vi "GUI_HTU_BCavePhosphors.vi"() -> ()   [LabVIEW 2020]
uses:
  Shared/GUI_Template/GUI_master/tcp_new_data_event.ctl
  Shared/GUI_Template/GUI_master/tcp new data cluster.ctl
  General GUIs/Device GUIs/GUI_Cameras/Controls/Crosshair type def.ctl
  <userlib>/_OpenG.lib/array/array.llb/Filter 1D Array with Scalar (String)__ogtk.vi
panel:
  in  "GUIdevice 8":string="U_PLC"
  in  "Position.Channel 8::7":T1(ring) caption="TC phosphor"
  in  "GUIdevice 7":string="U_1WireBcave"
  in  "DO.Ch4::8":enum16{"on", "off"}(ring) caption="Phosphor1"
  in  "DO.Ch2::8":enum16{"on", "off"}(ring) caption="Chicane Slits"
  in  "DigitalOutput.Channel 1::6":enum16{"on", "off"}(ring) caption="DC Phosphor"
  in  "GUIdevice 6":string="U_Valve_Daq"
  out "String 4":string="x1\ny1\nx2\ny2"
  out "String 3":string="x1\ny1\nx2\ny2"
  out "String 2":string="x1\ny1\nx2\ny2"
  out "String":string="x1\ny1\nx2\ny2"
  in  "visibility":bool=TRUE
  out "appended array":string[](array[string]) caption="XH"
  out "appended array 6":string[](array[string]) caption="XH"
  out "appended array 8":string[](array[string]) caption="XH"
  out "appended array 4":string[](array[string]) caption="XH"
  in  "UDP error message":string
  out "tcp data event 2":T2
  out "error IO 2":errorcluster
  in  "Color Box":u32(colorbox)
  in  "TargetSize.Y::5":dbl=45.0 caption="y" min=2.0 max=3000.0 format="%#_6f"
  in  "TargetSize.X::5":dbl=47.0 caption="x" min=2.0 max=3000.0 format="%#_6f"
  in  "TargetSize.Y::4":dbl=45.0 caption="y" min=2.0 max=3000.0 format="%#_6f"
  in  "TargetSize.X::4":dbl=47.0 caption="x" min=2.0 max=3000.0 format="%#_6f"
  in  "TargetSize.Y::3":dbl=163.0 caption="y" min=2.0 max=3000.0 format="%#_6f"
  in  "TargetSize.X::3":dbl=152.0 caption="x" min=2.0 max=3000.0 format="%#_6f"
  in  "TargetSize.Y::2":dbl=74.0 caption="y" min=2.0 max=3000.0 format="%#_6f"
  in  "TargetSize.X::2":dbl=75.0 caption="x" min=2.0 max=3000.0 format="%#_6f"
  in  "active cams":string
  out "CCDs":string[](array[string])
  out "Cameras":T3
  in  "Target.Y::5":dbl=45.0 caption="y" min=0.0 max=2000.0 format="%#_6f"
  in  "Target.X::5":dbl=47.0 caption="x" min=0.0 max=2000.0 format="%#_6f"
  in  "Target.Y::4":dbl=45.0 caption="y" min=0.0 max=2000.0 format="%#_6f"
  in  "Target.X::4":dbl=47.0 caption="x" min=0.0 max=2000.0 format="%#_6f"
  in  "Target.Y::3":dbl=163.0 caption="y" min=0.0 max=2000.0 format="%#_6f"
  in  "Target.X::3":dbl=152.0 caption="x" min=0.0 max=2000.0 format="%#_6f"
  in  "Target.Y::2":dbl=74.0 caption="y" min=0.0 max=2000.0 format="%#_6f"
  in  "Target.X::2":dbl=75.0 caption="x" min=0.0 max=2000.0 format="%#_6f"
  out "error out":errorcluster
  in  "triggerdelay::5":dbl=0.001 caption="triggerdelay" min=0.0 max=50000.0 format="%_4p"
  in  "triggerdelay::4":dbl=0.001 caption="triggerdelay" min=0.0 max=50000.0 format="%_4p"
  in  "triggerdelay::3":dbl=0.001 caption="triggerdelay" min=15.0 max=1000000.0 format="%_4p"
  in  "triggerdelay::2":dbl=0.001 caption="triggerdelay" min=500.0 max=1000000.0 format="%_4p"
  in  "trigger::5":bool caption="Trigger"
  in  "centroidy::5":dbl=0.001 caption="centroid y" min=0.0 max=0.0 format="%_4f"
  in  "centroidx::5":dbl=0.001 caption="centroid x" min=0.0 max=0.0 format="%_4f"
  in  "exposure::5":dbl=0.001 caption="exposure" min=0.0001 max=1.0 format="%_4p"
  out "image::5":T4(plugin-control) caption="HTT-MagCam-01"
  in  "GUIdevice 5":string="UC_Phosphor1"
  in  "trigger::4":bool caption="Trigger"
  in  "centroidy::4":dbl=0.001 caption="centroid y" min=0.0 max=0.0 format="%_4f"
  in  "centroidx::4":dbl=0.001 caption="centroid x" min=0.0 max=0.0 format="%_4f"
  in  "exposure::4":dbl=0.001 caption="exposure" min=0.0001 max=1.0 format="%_4p"
  out "image::4":T4(plugin-control) caption="HTT-MagCam-02"
  in  "GUIdevice 4":string="UC_DiagnosticsPhosphor"
  in  "trigger::3":bool caption="Trigger"
  in  "centroidy::3":dbl=0.001 caption="centroid y" min=0.0 max=0.0 format="%_4f"
  in  "centroidx::3":dbl=0.001 caption="centroid x" min=0.0 max=0.0 format="%_4f"
  in  "exposure::3":dbl=0.001 caption="exposure" min=2e-05 max=1.0 format="%_4p"
  out "image::3":T4(plugin-control) caption="HTT-MagCam-03"
  in  "GUIdevice 3":string="UC_ChicaneSlit"
  in  "trigger::2":bool caption="Trigger"
  in  "centroidy::2":dbl=0.001 caption="centroid y" min=0.0 max=0.0 format="%_4f"
  in  "centroidx::2":dbl=0.001 caption="centroid x" min=0.0 max=0.0 format="%_4f"
  in  "exposure::2":dbl=0.001 caption="exposure" min=2e-05 max=1.0 format="%_4p"
  out "image::2":T4(plugin-control) caption="HTT-MagCam-04"
  in  "GUIdevice 2":string="UC_TC_Phosphor"
  out "tcp data event":T2
  in  "Refresh Button":bool caption="Update Crosshairs"
  in  "Select device":string(combo)="FrogHPD"
  in  "stop":bool
  in  "GUIdevice 1":string="HPD_CCD"
  # "XHair location"
  # "XHair location"
  # "XHair size"
  # "XHair size"
  # "XHair location"
  # "XHair size"
  # "XHair size"
  # "XHair location"
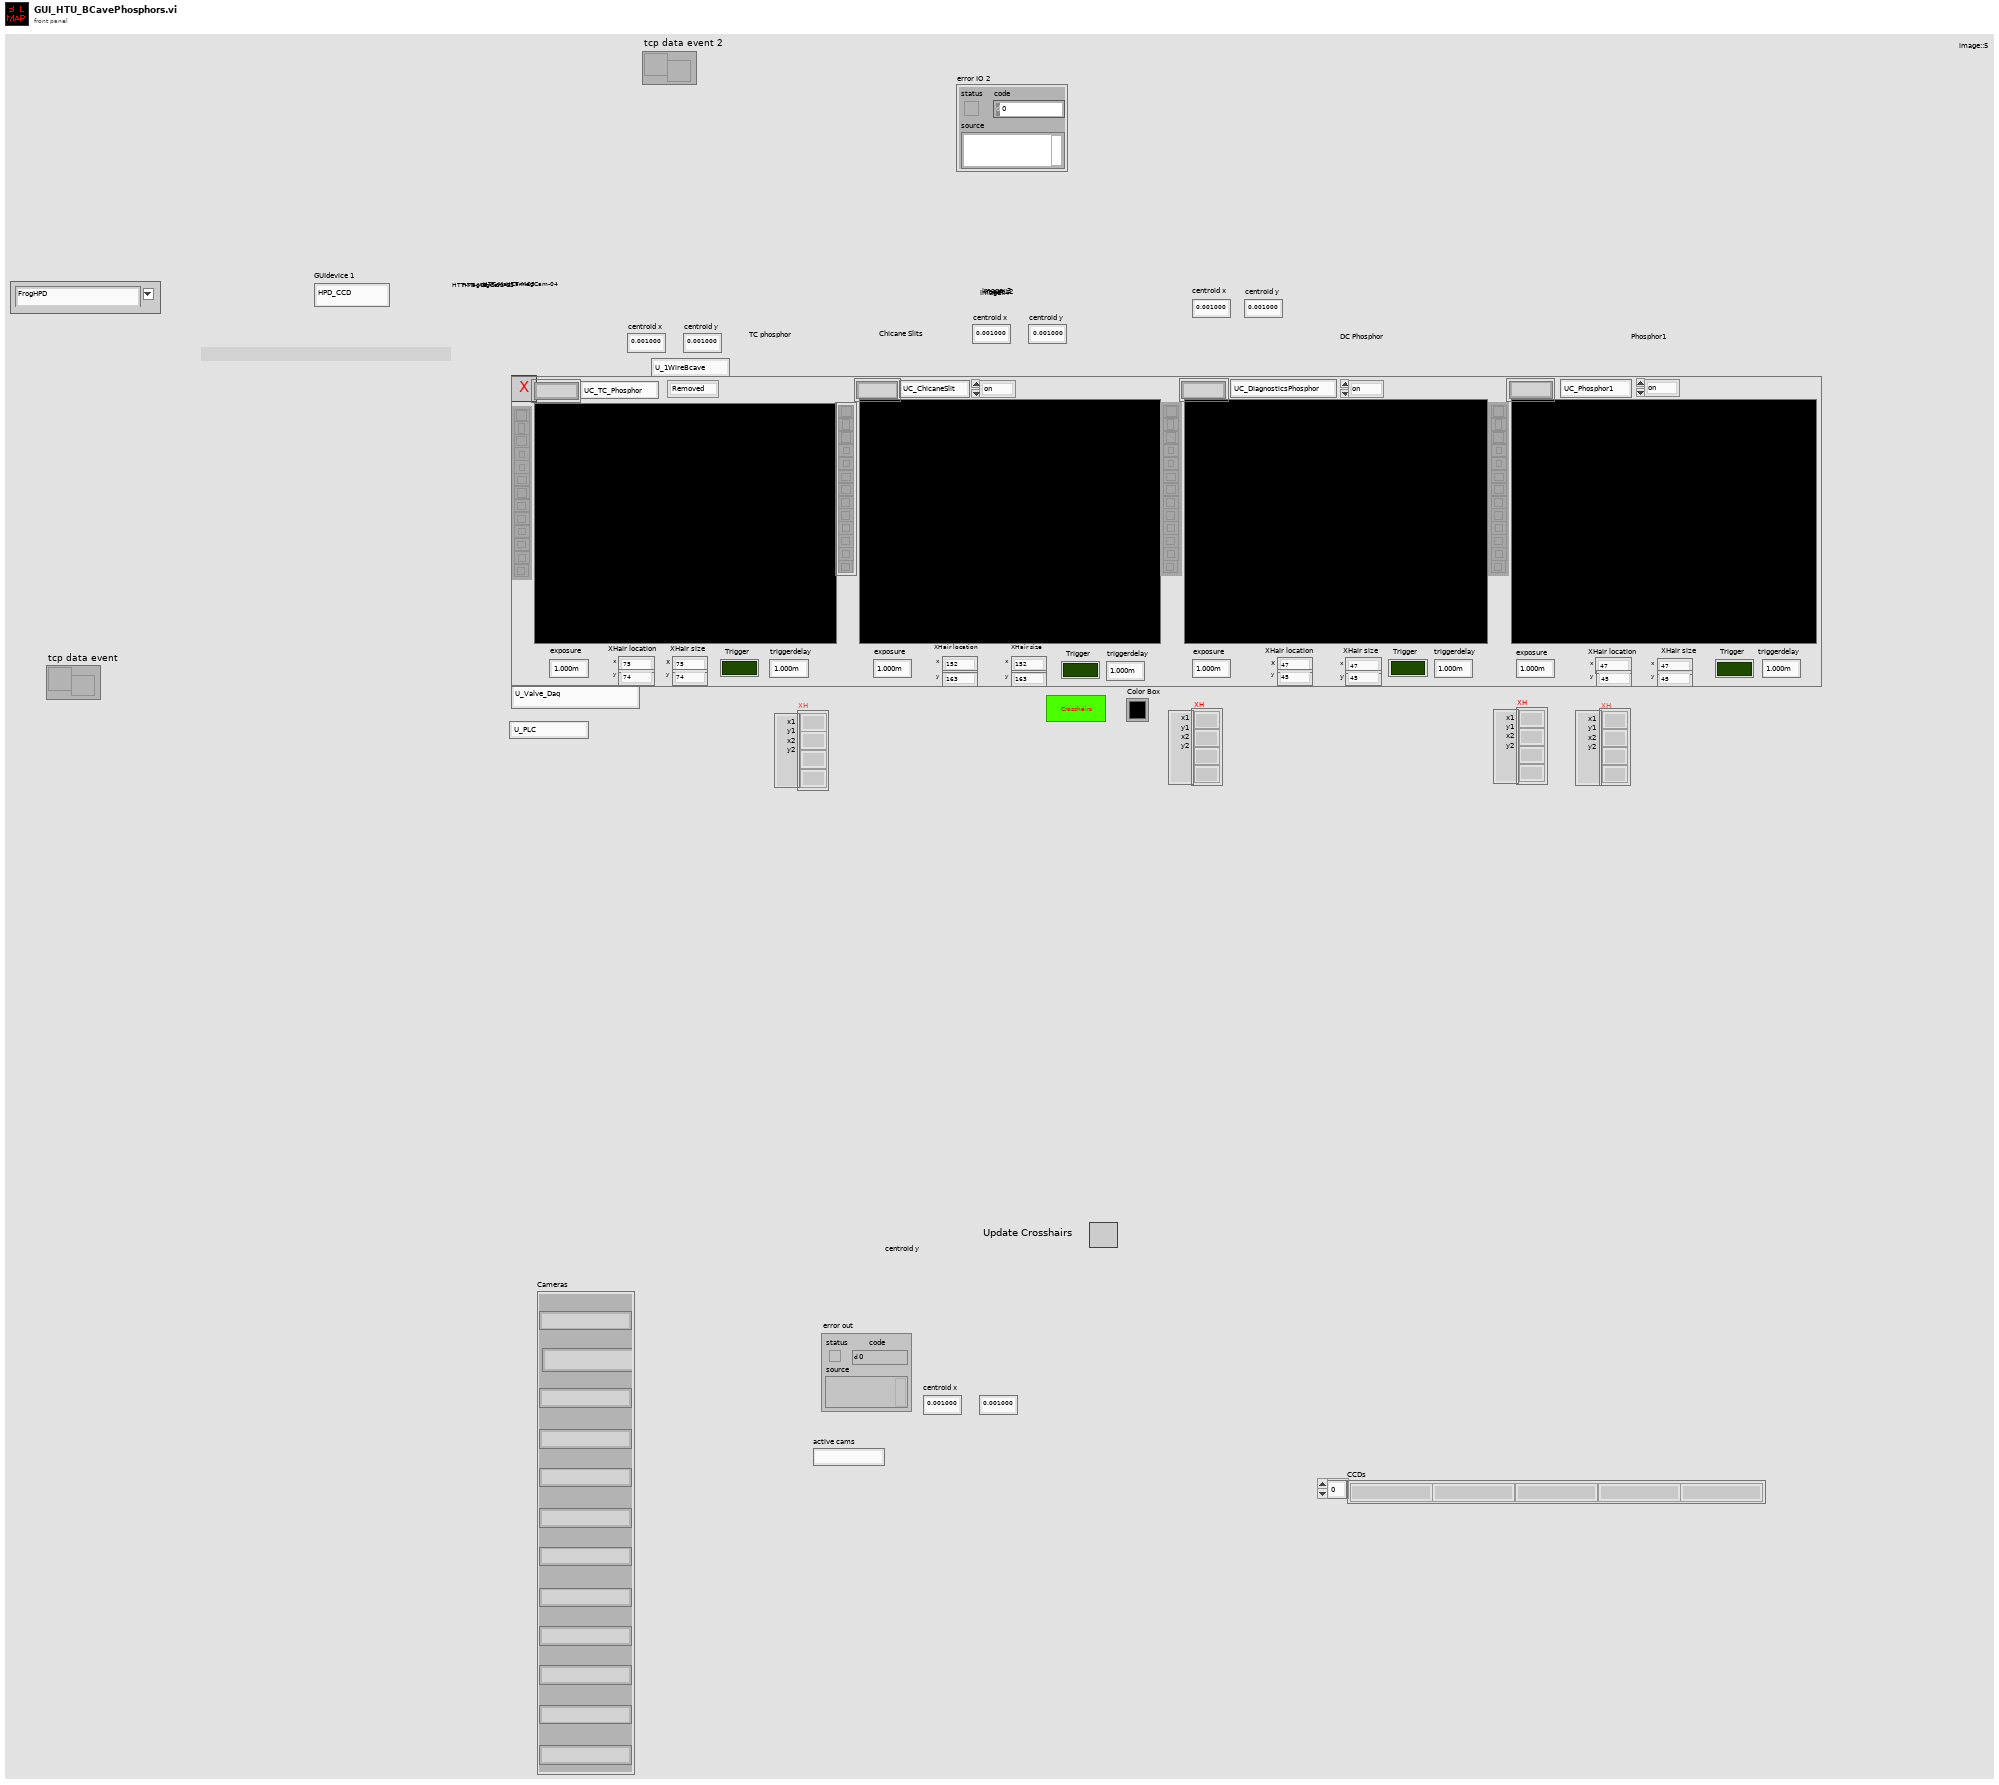
[diagram p1: front panel]
types:
  T1 = enum16{"Removed", "Inserted", "Unknown", "Moving"}
  T2 = typedef "tcp_new_data_event.ctl" = refnum<user-event>
  T3 = cluster{"[0]":string, "[1]":string, "[2]":string, "[3]":string, "[4]":string, "[5]":string, "[6]":string, "[7]":string, "[8]":string, "[8] 2":string, "[8] 3":string, "[8] 4":string}
  T4 = typedef "IMAQ Image.ctl" = refnum<image>
  T5 = typedef "Image Type" = u32
  T6 = cluster{"Target.X::2":refnum<vi>, "Target.Y::2":refnum<vi>}
  T7 = cluster{"Target.X::3":refnum<vi>, "Target.Y::3":refnum<vi>}
  T8 = cluster{"Target.X::4":refnum<vi>, "Target.Y::4":refnum<vi>}
  T9 = cluster{"Target.X::5":refnum<vi>, "Target.Y::5":refnum<vi>}
  T10 = cluster{"TargetSize.X::2":refnum<vi>, "TargetSize.Y::2":refnum<vi>}
  T11 = cluster{"TargetSize.X::3":refnum<vi>, "TargetSize.Y::3":refnum<vi>}
  T12 = cluster{"TargetSize.X::4":refnum<vi>, "TargetSize.Y::4":refnum<vi>}
  T13 = cluster{"TargetSize.X::5":refnum<vi>, "TargetSize.Y::5":refnum<vi>}
  T14 = cluster{"Target.X::5":refnum<vi>, "Target.Y::5":refnum<vi>}[]
  T15 = cluster{"TargetSize.X::5":refnum<vi>, "TargetSize.Y::5":refnum<vi>}[]
  T16 = cluster{"[0]":string, "[1]":string, "[2]":string, "[3]":string, "[4]":string, "[5]":string, "[6]":string, "[7]":string, "[8]":string, "[9]":string, "[10]":string, "[11]":string}
  T17 = typedef "Crosshair type def.ctl" = cluster{"Draw":bool, "Target":cluster{"x":dbl, "y":dbl}, "Size":cluster{"x":dbl, "y":dbl}, "Angle":dbl, "Color":u32, "Thickness":u8, "CrosshairLabel":string}
  T18 = cluster{"Left":i32, "Top":i32, "Right":i32, "Bottom":i32}
  T19 = enum32{"invalid app kind", "Development System", "Run Time System", "Student Edition", "Embedded LabVIEW", "Evaluation", "Custom"}
  T20 = typedef "tcp new data cluster.ctl" = cluster{"EventEnum":enum16{"new data", "connection status update"}, "Device name":string}
  T21 = enum32{"Invalid", "Standard", "Closed", "Hidden", "Minimized", "Maximized"}
  T22 = cluster{"Core":cluster{"Current VI Reference":refnum<vi>, "Close Panel on Exit?":bool}, "Your Boolean data":bool, "active cams":string, "SuperGUI":cluster{"STOP queue":refnum<queue>, "SuperGUI ref":refnum<vi>}}
  T23 = cluster{"STOP queue":refnum<queue>, "SuperGUI ref":refnum<vi>}
  T24 = cluster{"Current VI Reference":refnum<vi>, "Close Panel on Exit?":bool}
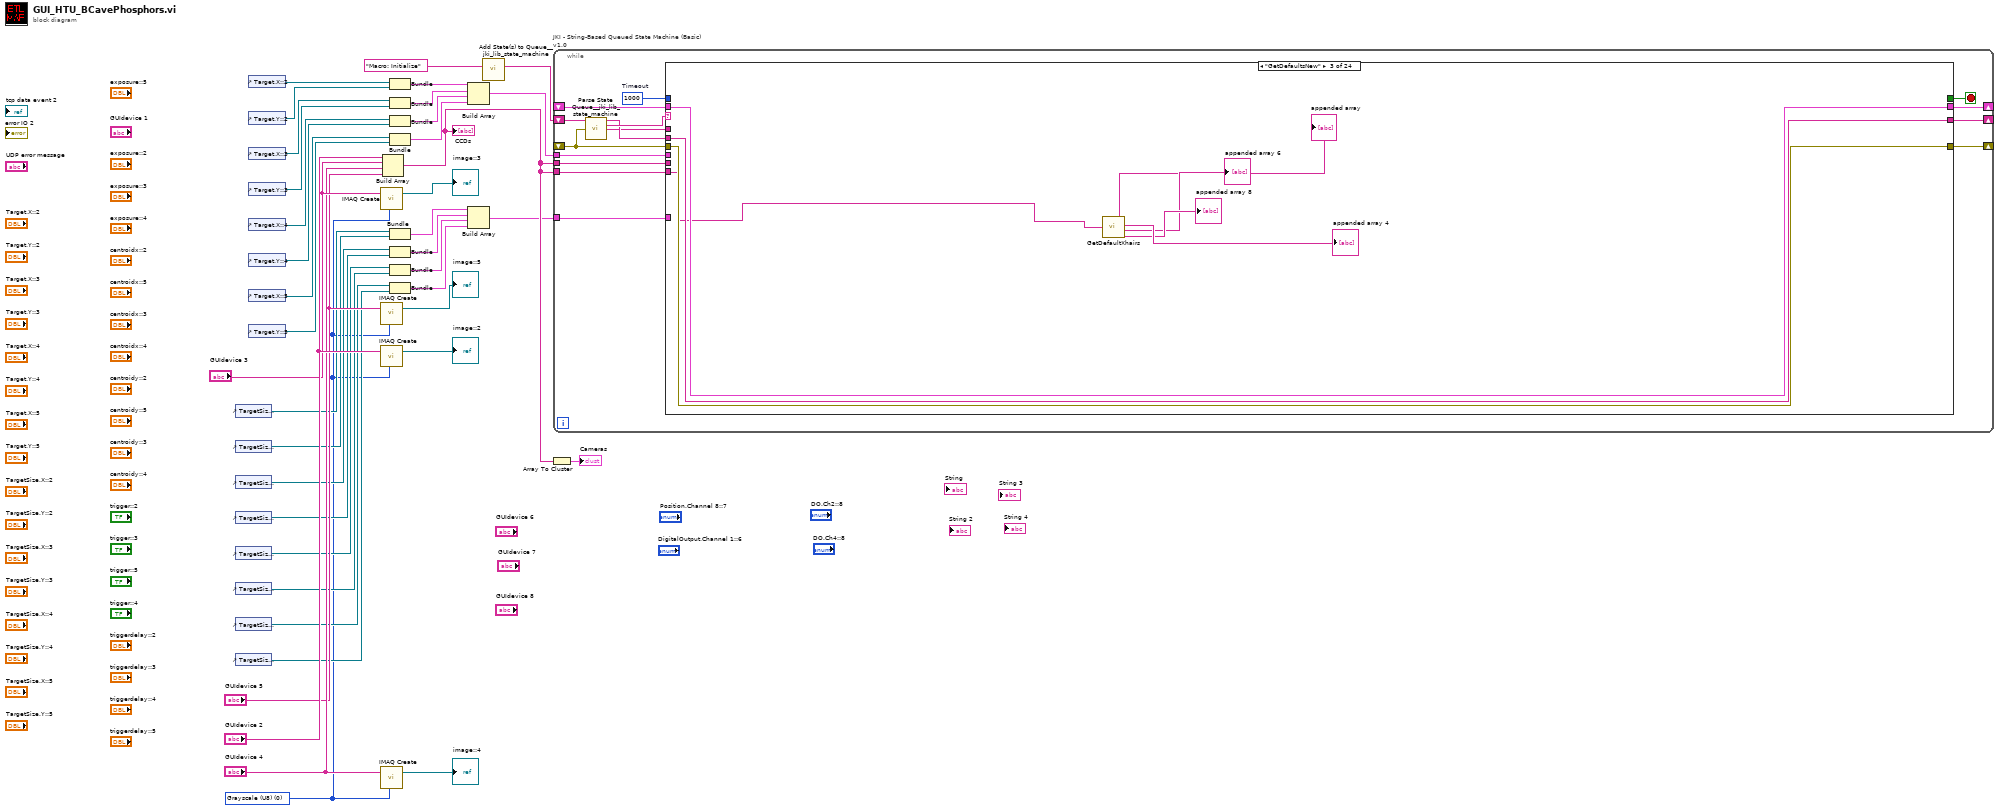
[diagram p0: block diagram]
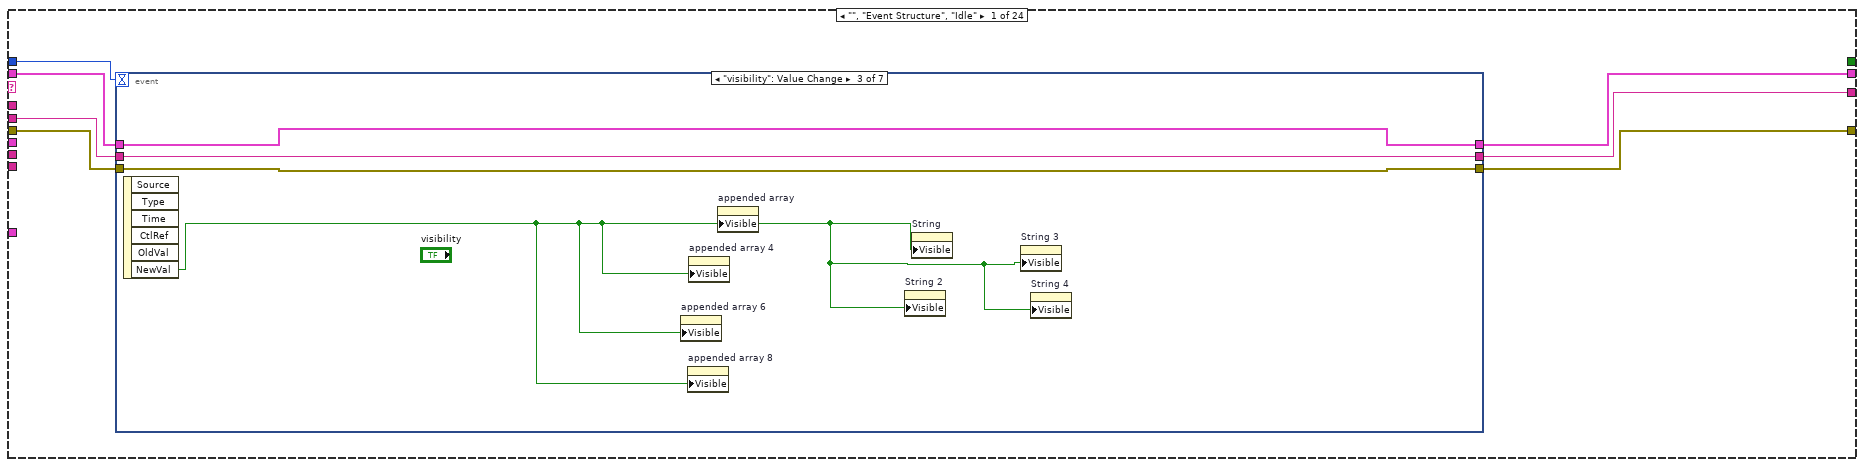
[diagram p2: hidden frame]
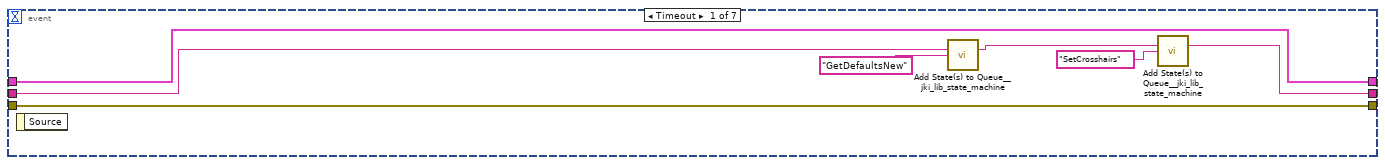
[diagram p3: hidden frame]
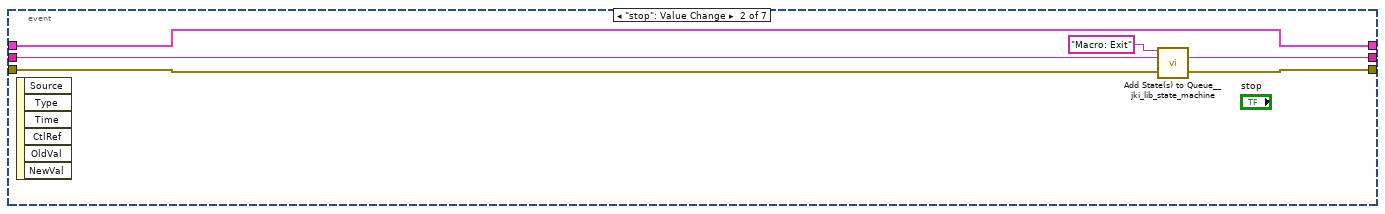
[diagram p4: hidden frame]
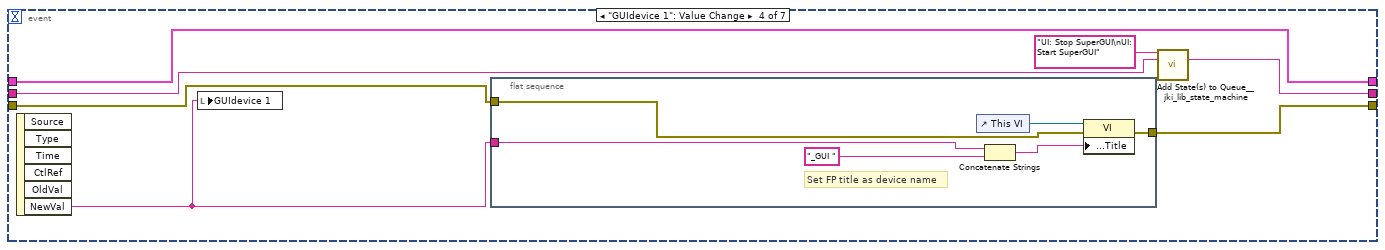
[diagram p5: hidden frame]
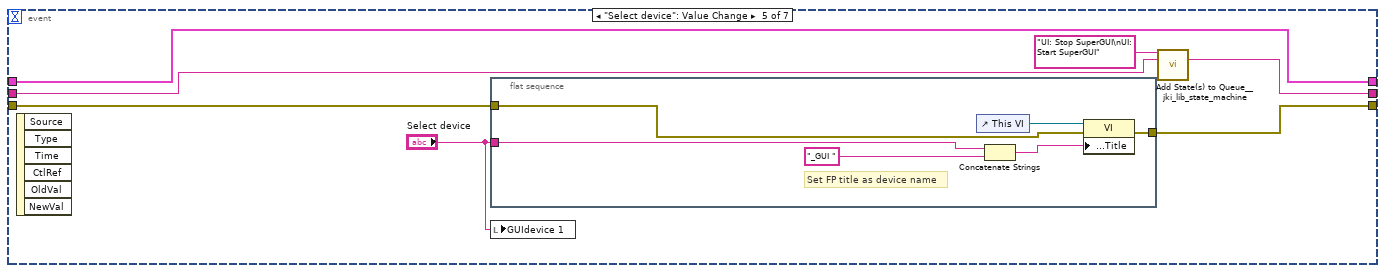
[diagram p6: hidden frame]
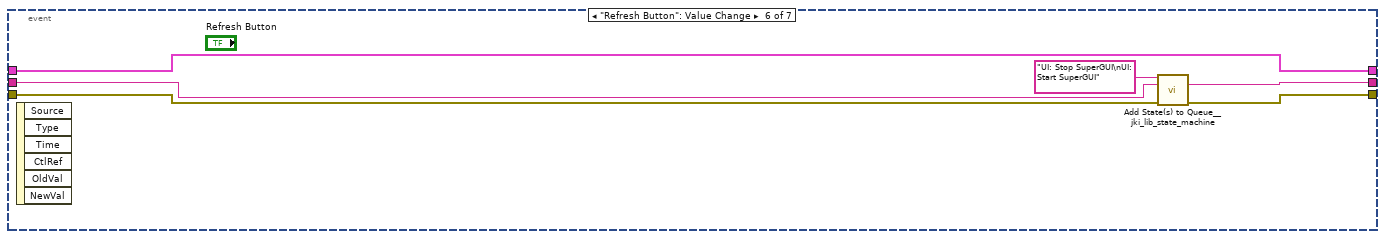
[diagram p7: hidden frame]
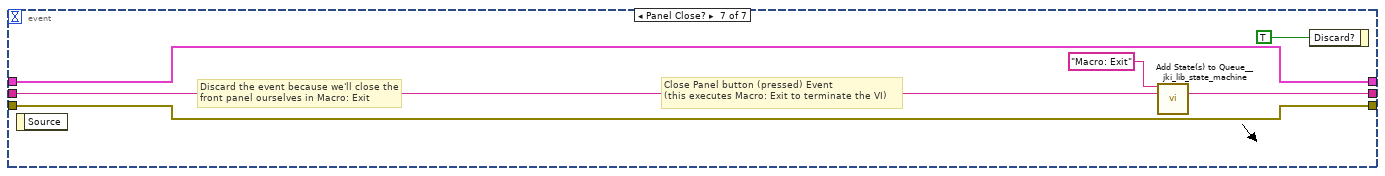
[diagram p8: hidden frame]
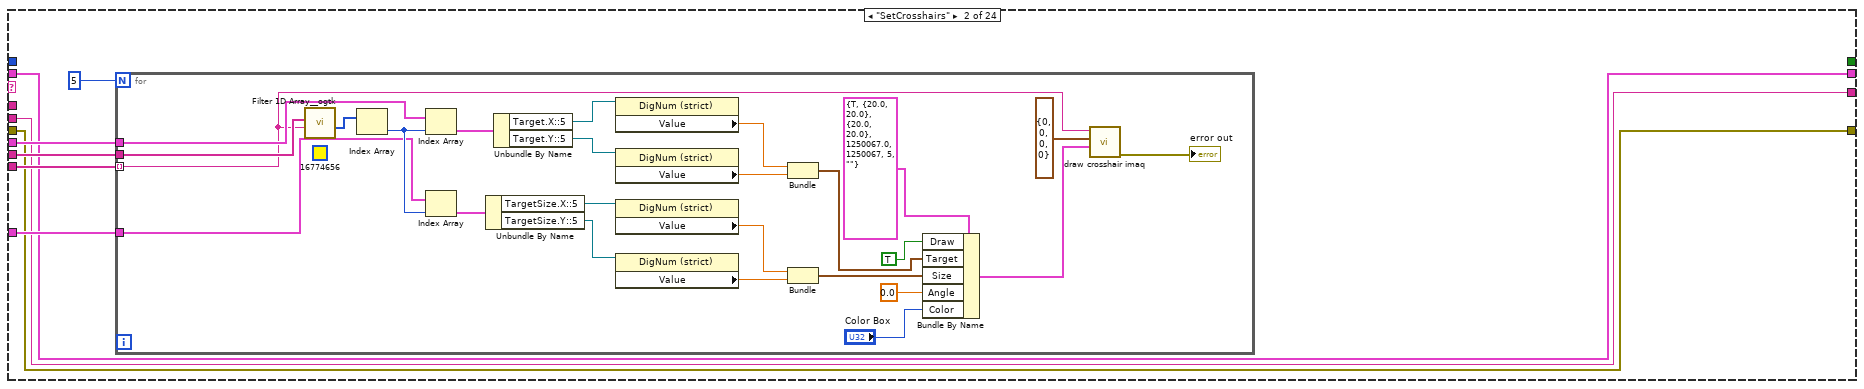
[diagram p9: hidden frame]
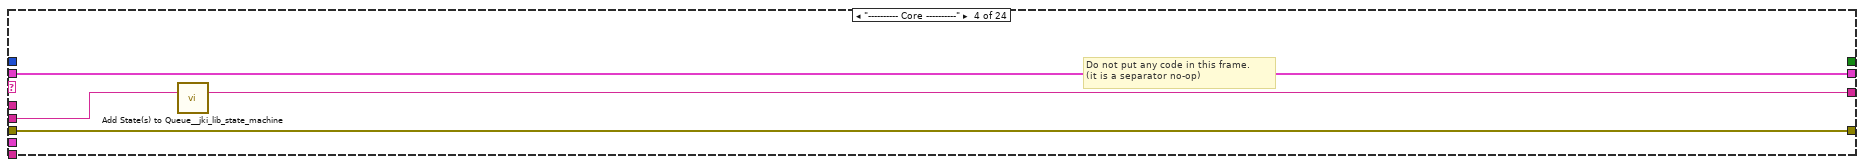
[diagram p10: hidden frame]
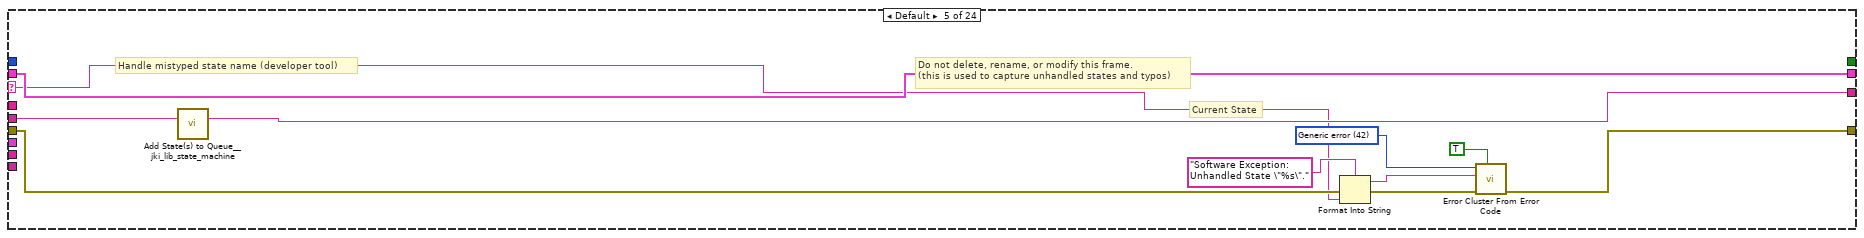
[diagram p11: hidden frame]
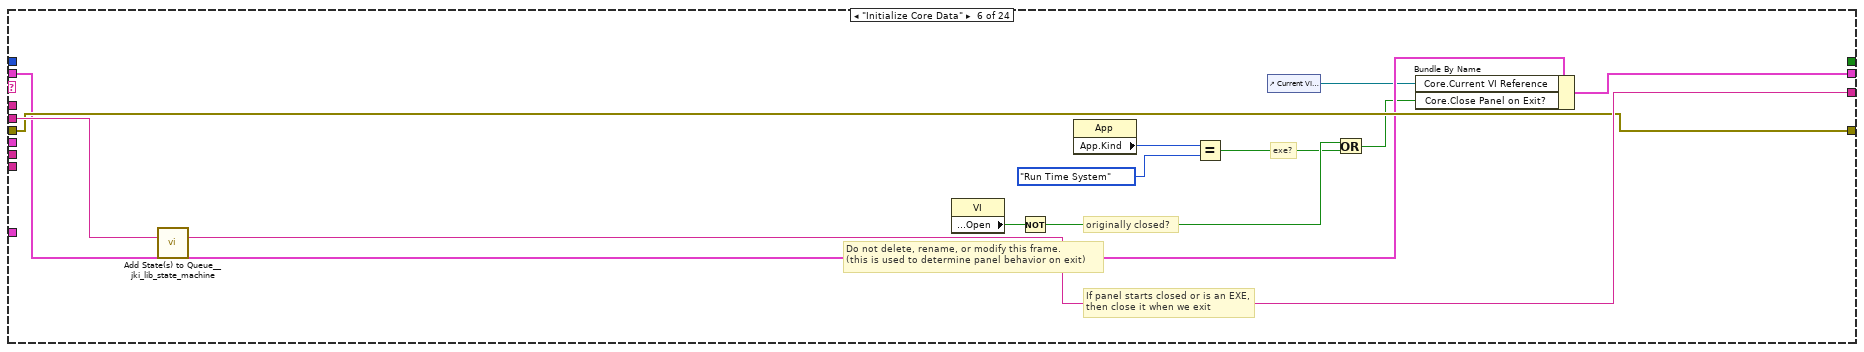
[diagram p12: hidden frame]
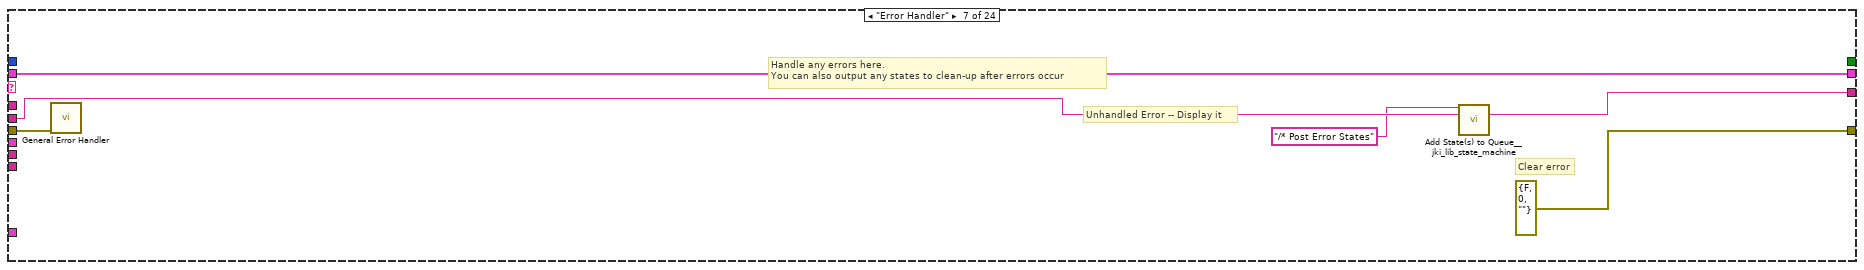
[diagram p13: hidden frame]
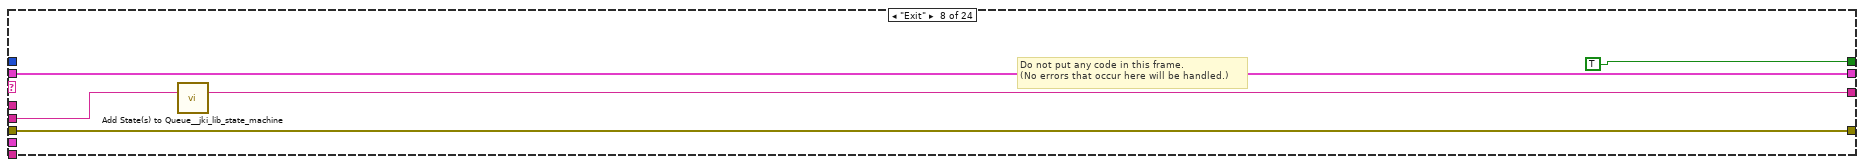
[diagram p14: hidden frame]
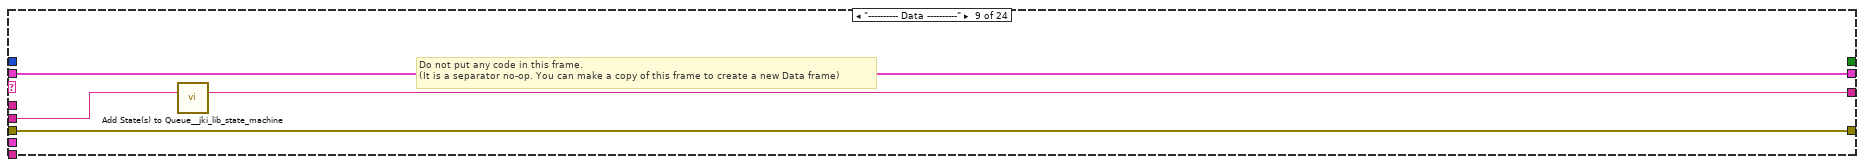
[diagram p15: hidden frame]
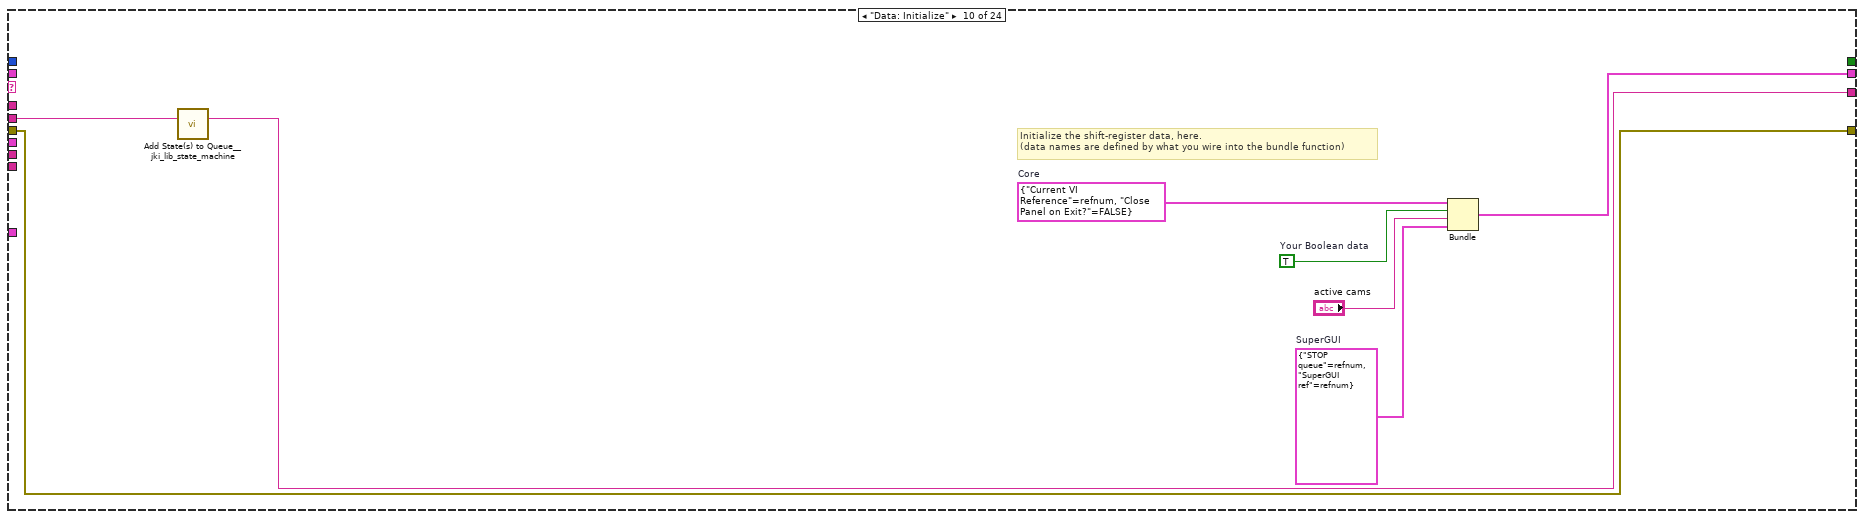
[diagram p16: hidden frame]
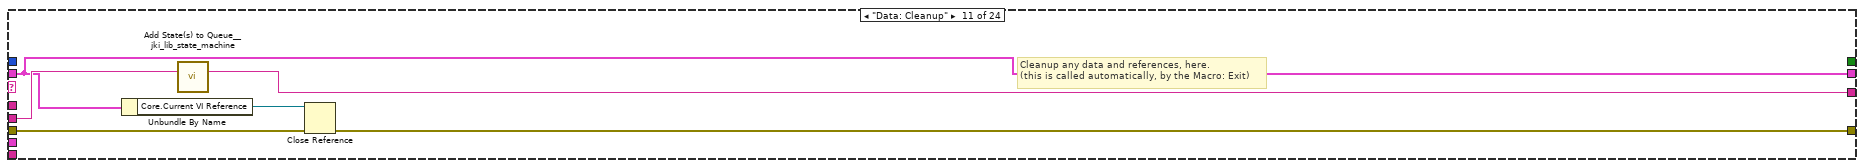
[diagram p17: hidden frame]
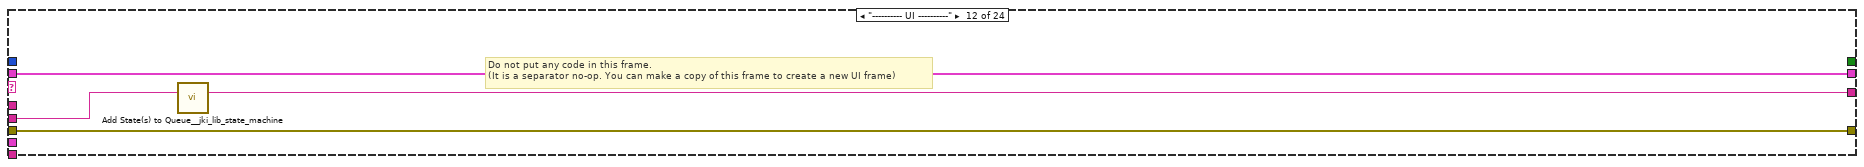
[diagram p18: hidden frame]
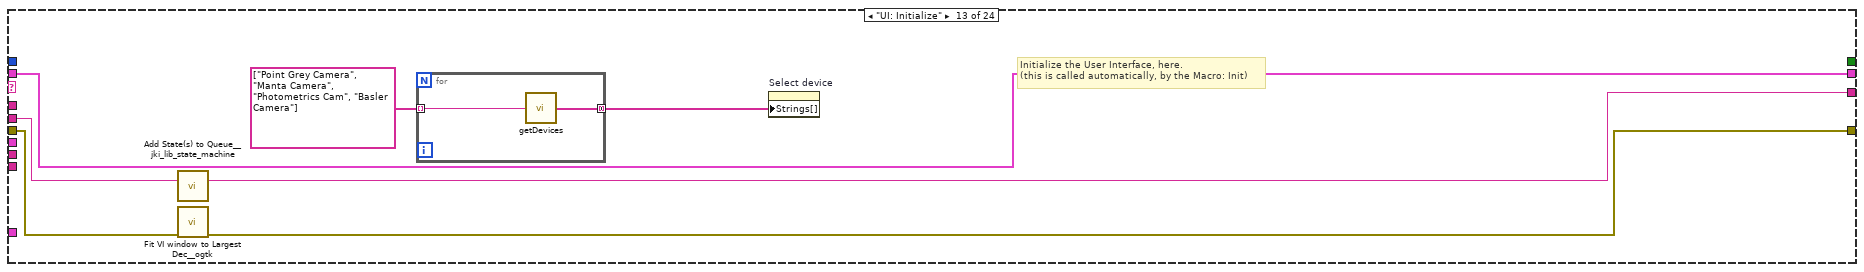
[diagram p19: hidden frame]
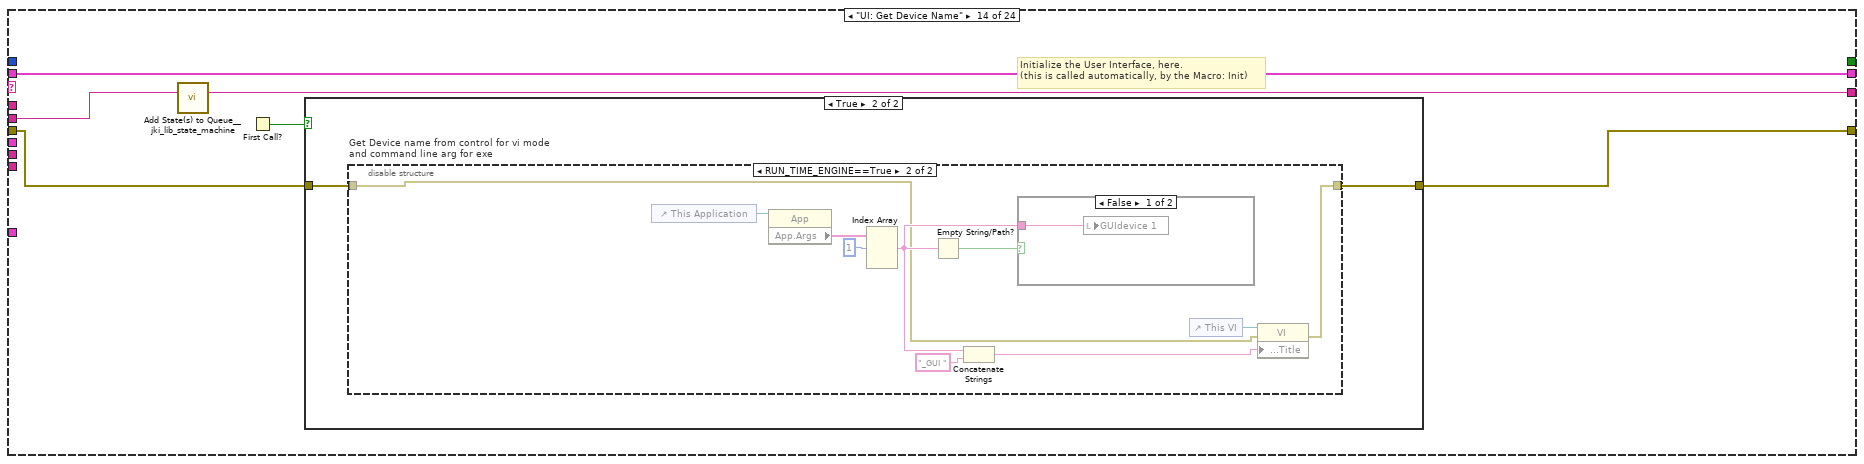
[diagram p20: hidden frame]
diagram:
  w1 = T5 0 items=["Grayscale (U8)", "Grayscale (I16)", "Grayscale (SGL)", "Complex (CSG)", "RGB (U32)", "HSL (U32)", "RGB (U64)", "Grayscale (U16)"] ("Image Type")
  n1 = control-ref of="TargetSize.X::2"() -> (w14:refnum<vi>)
  n2 = control-ref of="TargetSize.Y::2"() -> (w13:refnum<vi>)
  n3 = control-ref of="TargetSize.X::3"() -> (w12:refnum<vi>)
  n4 = control-ref of="TargetSize.Y::3"() -> (w11:refnum<vi>)
  n5 = control-ref of="TargetSize.X::4"() -> (w10:refnum<vi>)
  n6 = control-ref of="TargetSize.Y::4"() -> (w9:refnum<vi>)
  n7 = control-ref of="TargetSize.X::5"() -> (w8:refnum<vi>)
  n8 = control-ref of="TargetSize.Y::5"() -> (w7:refnum<vi>)
  n9 = control-ref of="Target.X::2"() -> (w33:refnum<vi>)
  n10 = control-ref of="Target.Y::2"() -> (w32:refnum<vi>)
  n11 = control-ref of="Target.X::3"() -> (w31:refnum<vi>)
  n12 = control-ref of="Target.Y::3"() -> (w30:refnum<vi>)
  n13 = control-ref of="Target.X::4"() -> (w29:refnum<vi>)
  n14 = control-ref of="Target.Y::4"() -> (w28:refnum<vi>)
  n15 = control-ref of="Target.X::5"() -> (w27:refnum<vi>)
  n16 = control-ref of="Target.Y::5"() -> (w26:refnum<vi>)
  n17 = call "IMAQ Create"("Image Name"="GUIdevice 3", "Image Type"=w1) -> ("New Image"=→"image::3":T4)  [unwired: 3 in, 1 out]
  n18 = call "IMAQ Create"("Image Name"="GUIdevice 5", "Image Type"=w1) -> ("New Image"=→"image::5":T4)  [unwired: 3 in, 1 out]
  n19 = call "IMAQ Create"("Image Name"="GUIdevice 2", "Image Type"=w1) -> ("New Image"=→"image::2":T4)  [unwired: 3 in, 1 out]
  n20 = call "IMAQ Create"("Image Name"="GUIdevice 4", "Image Type"=w1) -> ("New Image"=→"image::4":T4)  [unwired: 3 in, 1 out]
  n21 = Build Array("GUIdevice 2", "GUIdevice 3", "GUIdevice 4", "GUIdevice 5") -> (w15:string[])
  "CCDs" <- w15
  n22 = Bundle("Target.X::2"=w33, "Target.Y::2"=w32) -> (w25:T6)  [unwired: 1 in]
  n23 = Bundle("Target.X::3"=w31, "Target.Y::3"=w30) -> (w24:T7)  [unwired: 1 in]
  n24 = Bundle("Target.X::4"=w29, "Target.Y::4"=w28) -> (w22:T8)  [unwired: 1 in]
  n25 = Bundle("Target.X::5"=w27, "Target.Y::5"=w26) -> (w23:T9)  [unwired: 1 in]
  n26 = Bundle("TargetSize.X::2"=w14, "TargetSize.Y::2"=w13) -> (w6:T10)  [unwired: 1 in]
  n27 = Bundle("TargetSize.X::3"=w12, "TargetSize.Y::3"=w11) -> (w5:T11)  [unwired: 1 in]
  n28 = Bundle("TargetSize.X::4"=w10, "TargetSize.Y::4"=w9) -> (w3:T12)  [unwired: 1 in]
  n29 = Bundle("TargetSize.X::5"=w8, "TargetSize.Y::5"=w7) -> (w4:T13)  [unwired: 1 in]
  n30 = Build Array(w25, w24, w22, w23) -> (w21:T14)
  n31 = Build Array(w6, w5, w3, w4) -> (w2:T15)
  n32 = call <vilib>:"Add State(s) to Queue__jki_lib_state_machine.vi"("State(s) in (\"\")"="Macro: Initialize") -> ("States Out"=w39:string)  [unwired: 14 in]
  n33 = Array To Cluster(array=w15) -> (cluster=→"Cameras":T16)
  n34 = while "JKI - String-Based Queued State Machine (Basic) v1.0" {
    shift-right: [w47] -> _
    shift-left: _ -> [w44]
    shift-right: [w50] -> _
    shift-left: _ -> [w45]
    shift-right: [w49] -> _
    shift-left: w39 -> [w51]
    tunnel: w21 -> [w41]
    tunnel: w15 -> [w42]
    tunnel: w15 -> [w43]
    tunnel: w2 -> [w40]
    stop <- w48 stop-if-true
    w46 = 1000  # Timeout
    n35 = call <vilib>:"Parse State Queue__jki_lib_state_machine.vi"("State Queue"=w51, "Error In (no error)"=w45) -> ("Remaining States"=w53:string, "Current State"=w54:string, "Arguments"=w52:string)  [unwired: 11 in]
    n36 = case shown="\"GetDefaultsNew\"" w54 {
      selector: w54 -> [_ _ _ _ w160 _ _ _ _ _ _ _ _ _ _ _ _ _ _ _ _ _ _ _]
      tunnel: w53 -> [w61 w117 w154 w159 w164 w182 w188 w193 w197 w205 w211 w215 w222 w230 w265 w273 w279 w290 w316 w321 w331 w335 w339 w343]
      tunnel: w52 -> [_ _ _ _ _ _ _ _ _ _ _ _ _ _ _ _ w274 w284 _ _ _ _ _ _]
      tunnel: w44 -> [w59 w118 w155 w156 w162 w173 w185 w191 w194 _ w206 w212 w220 w228 w256 w268 w277 w286 w313 w318 w328 w332 w336 w340]
      tunnel: [w58 w116 w153 w157 w166 w179 errorcluster {"status"=FALSE, "code"=0, "source"=""} ("error out") w190 w195 w202 w207 w213 w218 w225 w249 w266 w275 w287 w314 w319 w329 w333 w337 w341] -> w50
      tunnel: w45 -> [w57 w116 w153 w157 w165 w179 w184 w190 w195 w202 w208 w213 w219 w226 w250 w267 w276 w288 w314 w319 w329 w333 w337 w341]
      tunnel: [w60 w117 w154 w158 w163 w181 w187 w192 w196 w204 w210 w214 w221 w229 w264 w272 w278 w289 w315 w320 w330 w334 w338 w342] -> w49
      tunnel: [_ _ _ _ _ _ _ TRUE _ _ _ _ _ _ _ _ _ _ _ _ _ _ _ _] -> w48
      tunnel: [w56 w118 w155 w156 w162 w180 w185 w191 w194 w203 w206 w212 w220 w228 w255 w268 w277 w286 w313 w318 w328 w332 w336 w340] -> w47
      tunnel: w46 -> [w55 _ _ _ _ _ _ _ _ _ _ _ _ _ _ _ _ _ _ _ _ _ _ _]
      tunnel: w43 -> [_ w120 w152 _ _ _ _ _ _ _ _ _ _ _ _ _ _ _ _ _ _ _ _ _]
      tunnel: w42 -> [_ w121 _ _ _ _ _ _ _ _ _ _ _ _ _ _ _ _ _ _ _ _ _ _]
      tunnel: w41 -> [_ w122 _ _ _ _ _ _ _ _ _ _ _ _ _ _ _ _ _ _ _ _ _ _]
      tunnel: w40 -> [_ w119 _ _ _ _ _ _ _ _ _ _ _ _ _ _ _ _ _ _ _ _ _ _]
      frame "", "Event Structure", "Idle" {
        n37 = event shown="[2] \"visibility\": Value Change" {
          selector: _ -> [_ _ _ _ _ _ _]
          dyn-events: _ -> [_ _ _ _ _ _ _]
          timeout: w55 -> [_ _ _ _ _ _ _]
          tunnel: w61 -> [w64 w71 w75 w81 w93 w106 w114]
          tunnel: [w68 w70 w75 w80 w92 w105 w113] -> w60
          tunnel: w59 -> [w66 w73 w77 w84 w97 w108 w111]
          tunnel: [w67 w72 w76 w82 w95 w107 w112] -> w58
          tunnel: w57 -> [w67 w72 w76 w83 w96 w107 w112]
          tunnel: [w66 w73 w77 w84 w97 w108 w111] -> w56
          event Timeout {
            n38 = event-data() -> ()  [unwired: 1 in, 1 out]
            n39 = call <vilib>:"Add State(s) to Queue__jki_lib_state_machine.vi"("State(s) in (\"\")"=w64, "State(s) at Back (\"\")"="GetDefaultsNew") -> ("States Out"=w62:string)  [unwired: 13 in]
            n40 = call <vilib>:"Add State(s) to Queue__jki_lib_state_machine.vi"("State(s) in (\"\")"=w62, "State(s) at Back (\"\")"="SetCrosshairs") -> ("States Out"=w68:string)  [unwired: 13 in]
          }
          event "stop": Value Change {
            n41 = event-data() -> ()  [unwired: 1 in, 6 out]
            n42 = call <vilib>:"Add State(s) to Queue__jki_lib_state_machine.vi"("State(s) in Front (\"\")"="Macro: Exit", "State(s) in (\"\")"=w71) -> ("States Out"=w70:string)  [unwired: 13 in]
          }
          event "visibility": Value Change {
            n43 = event-data() -> ("NewVal"=w74:bool)  [unwired: 1 in, 5 out]
            n44 = property on="appended array 6" class="Arr (strict)"("Visible"=w74) -> ()  [unwired: 2 in, 2 out]
            n45 = property on="appended array 8" class="Arr (strict)"("Visible"=w74) -> ()  [unwired: 2 in, 2 out]
            n46 = property on="appended array 4" class="Arr (strict)"("Visible"=w74) -> ()  [unwired: 2 in, 2 out]
            n47 = property on="appended array" class="Arr (strict)"("Visible"=w74) -> ()  [unwired: 2 in, 2 out]
            n48 = property on="String 2" class="Str"("Visible"=w74) -> ()  [unwired: 2 in, 2 out]
            n49 = property on="String" class="Str"("Visible"=w74) -> ()  [unwired: 2 in, 2 out]
            n50 = property on="String 3" class="Str"("Visible"=w74) -> ()  [unwired: 2 in, 2 out]
            n51 = property on="String 4" class="Str"("Visible"=w74) -> ()  [unwired: 2 in, 2 out]
          }
          event "GUIdevice 1": Value Change {
            n52 = event-data() -> ("NewVal"=w78:string)  [unwired: 1 in, 5 out]
            n53 = local write "GUIdevice 1"(w78) -> ()
            n54 = flat-sequence {
              tunnel: [w87] -> w82
              tunnel: w83 -> [w86]
              tunnel: w78 -> [w85]
              frame #0 {
                # "Set FP title as device name"
                n55 = control-ref of="This VI"() -> (w90:refnum<vi>)
                n56 = Concatenate Strings(w85, "_GUI ") -> (w89:string)
                n57 = property class="VI"(reference=w90, error in=w86, "Front Panel.Title"=w89) -> (error out=w87:errorcluster)  [unwired: 1 out]
              }
            }
            n58 = call <vilib>:"Add State(s) to Queue__jki_lib_state_machine.vi"("State(s) in Front (\"\")"="UI: Stop SuperGUI\nUI: Start SuperGUI", "State(s) in (\"\")"=w81) -> ("States Out"=w80:string)  [unwired: 13 in]
          }
          event "Select device": Value Change {
            n59 = event-data() -> ()  [unwired: 1 in, 6 out]
            n60 = flat-sequence {
              tunnel: [w100] -> w95
              tunnel: w96 -> [w99]
              tunnel: "Select device" -> [w98]
              frame #0 {
                # "Set FP title as device name"
                n61 = control-ref of="This VI"() -> (w103:refnum<vi>)
                n62 = Concatenate Strings(w98, "_GUI ") -> (w102:string)
                n63 = property class="VI"(reference=w103, error in=w99, "Front Panel.Title"=w102) -> (error out=w100:errorcluster)  [unwired: 1 out]
              }
            }
            n64 = local write "GUIdevice 1"("Select device") -> ()
            n65 = call <vilib>:"Add State(s) to Queue__jki_lib_state_machine.vi"("State(s) in Front (\"\")"="UI: Stop SuperGUI\nUI: Start SuperGUI", "State(s) in (\"\")"=w93) -> ("States Out"=w92:string)  [unwired: 13 in]
          }
          event "Refresh Button": Value Change {
            n66 = event-data() -> ()  [unwired: 1 in, 6 out]
            n67 = call <vilib>:"Add State(s) to Queue__jki_lib_state_machine.vi"("State(s) in Front (\"\")"="UI: Stop SuperGUI\nUI: Start SuperGUI", "State(s) in (\"\")"=w106) -> ("States Out"=w105:string)  [unwired: 13 in]
          }
          event Panel Close? {
            # "Discard the event because we'll close the front panel ourselves in Macro: Exit"
            # "Close Panel button (pressed) Event\n(this executes Macro: Exit to terminate the VI)"
            n68 = event-data() -> ()  [unwired: 1 in, 1 out]
            n69 = call <vilib>:"Add State(s) to Queue__jki_lib_state_machine.vi"("State(s) in Front (\"\")"="Macro: Exit", "State(s) in (\"\")"=w114) -> ("States Out"=w113:string)  [unwired: 13 in]
            n70 = event-data("Discard?"=TRUE) -> ()  [unwired: 1 in, 1 out]
          }
        }
      }
      frame "SetCrosshairs" {
        n71 = for {
          N: 5 -> [_]
          tunnel: w121 -> [w126]
          tunnel: w122 -> [w125]
          tunnel: w119 -> [w124]
          tunnel: w120 -> [w123] mode=indexing
          (unwired) u32 16774656 ("Color")
          n72 = call-poly <userlib>:"Filter 1D Array__ogtk.vi"("items to filter"=w123, "array"=w126) -> ("filtered item indices"=w130:i32[])  [unwired: 4 in, 1 out]
          n73 = Index Array(array=w130) -> (element=w133:i32)  [unwired: 1 in]
          n74 = Index Array(array=w125, index=w133) -> (element=w131:T9)
          n75 = Index Array(array=w124, index=w133) -> (element=w134:T13)
          n76 = Unbundle By Name(w134) -> ("TargetSize.X::5"=w135:refnum<vi>, "TargetSize.Y::5"=w136:refnum<vi>)
          n77 = Unbundle By Name(w131) -> ("Target.X::5"=w128:refnum<vi>, "Target.Y::5"=w129:refnum<vi>)
          n78 = property class="DigNum (strict)"(reference=w128) -> ("Value"=w142:dbl)  [unwired: 1 in, 2 out]
          n79 = property class="DigNum (strict)"(reference=w129) -> ("Value"=w143:dbl)  [unwired: 1 in, 2 out]
          n80 = property class="DigNum (strict)"(reference=w135) -> ("Value"=w137:dbl)  [unwired: 1 in, 2 out]
          n81 = property class="DigNum (strict)"(reference=w136) -> ("Value"=w138:dbl)  [unwired: 1 in, 2 out]
          n82 = Bundle("Value"=w142, "Value"=w143) -> (w144:cluster{"Value":dbl, "Value":dbl})  [unwired: 1 in]
          n83 = Bundle("Value"=w137, "Value"=w138) -> (w145:cluster{"Value":dbl, "Value":dbl})  [unwired: 1 in]
          n84 = Bundle By Name(cluster=T17 {"Draw"=TRUE, "Target"={"x"=20.0, "y"=20.0}, "Size"={"x"=20.0, "y"=20.0}, "Angle"=1250067.0, "Color"=1250067, "Thickness"=5, "CrosshairLabel"=""} ("Crosshair"), "Draw"=TRUE, "Target"=w144, "Size"=w145, "Angle"=0.0, "Color"="Color Box") -> (w140:T17)
          n85 = call "draw crosshair imaq.vi"("Crosshair"=w140, "Bounding Rectangle"=T18 {"Left"=0, "Top"=0, "Right"=0, "Bottom"=0}, "image in"=w123) -> ("error out"=→"error out":errorcluster)  [unwired: 7 in, 1 out]
        }
      }
      frame "GetDefaultsNew" {
        n86 = call "GetDefaultXhairs.vi"("appended array 2"=w152) -> ("appended array"=→"appended array":string[], "appended array 4"=→"appended array 4":string[], "appended array 6"=→"appended array 6":string[], "appended array 8"=→"appended array 8":string[])
      }
      frame "---------- Core ----------" {
        # "Do not put any code in this frame.\n(it is a separator no-op)"
        n87 = call <vilib>:"Add State(s) to Queue__jki_lib_state_machine.vi"("State(s) in (\"\")"=w159) -> ("States Out"=w158:string)  [unwired: 14 in]
      }
      frame Default {
        w169 = 42 items=["No error", "Argument error", "Memory is full", "Out of zone", "End of file", "File already open", "Generic file I/O error", "File not found", "File permission error", "Disk is full", "Duplicate path", "Too many files open", "System feature not enabled", "Resource file not found", "Cannot add resource", "Resource not found", "Image not found", "Image memory error", "Pen does not exist", "Config type invalid", "Config token not found", "Config parse error", "Config memory error", "Bad external code format", "Bad external code offset", "External code not present", "Null window", "Destroy window error", "Null menu", "Print aborted", "Bad print record", "Print driver error", "Windows error during printing", "Memory error during printing", "Print dialog error", "Generic print error", "Invalid device refnum", "Device not found", "Device parameter error", "Device unit error", "Cannot open device", "Device call aborted", "Generic error", "Cancelled by user", "Object ID too low", "Object ID too high", "Object not in heap", "Unknown heap", "Unknown object (invalid DefProc)", "Unknown object (DefProc not in table)", "Message out of range", "Invalid (null) method", "Unknown message", "Manager call not supported", "Bad address", "Network operation in progress", "Network operation timed out", "Connection is busy", "Network attribute not supported", "Network error", "Address in use", "System out of memory", "Connection aborted", "Connection refused", "Not connected", "Already connected", "Connection closed", "Initialization error (interapplication manager)", "Bad occurrence", "Wait on unbound occurrence handler", "Occurrence queue overflow", "Datalog type conflict", "Unused", "Unrecognized type (interapplication manager)", "Memory corrupt", "Failed to make temporary DLL", "Old CIN version", "Drag socket not found", "Failed to load drop-object", "Failed to register OLE object", "Failed to release OLE object", "Format specifier type mismatch", "Unknown format specifier", "Too few format specifiers", "Too many format specifiers", "Scan failed", "Newer CIN version", "Error converting to variant", "Runtime menu error", "Password tampered", "Variant attribute not found", "Incompatible variant data type", "Event data is not available", "Event Store is not present", "Occurrence is not found", "Event Queue is not created", "Event info is not available", "Refnum passed is NULL", "Error retrieving Class GUID", "Error retrieving CoClass GUID", "Error retrieving TypeLib GUID.", "Bad built application magic bytes.", "Specific driver is different from the specific driver associated with the Logical Name.", "There is no session opened to the class driver.", "Max Error", "MAX - Error with config objects", "MAX - Error loading configuration", "MAX - Group not supported"]
        # "Current State"
        # "Do not delete, rename, or modify this frame.\n(this is used to capture unhandled states and typos)"
        # "Handle mistyped state name (developer tool)"
        n88 = call <vilib>:"Add State(s) to Queue__jki_lib_state_machine.vi"("State(s) in (\"\")"=w164) -> ("States Out"=w163:string)  [unwired: 14 in]
        n89 = Format Into String(format string="Software Exception: Unhandled State \"%s\"." ("message"), error in=w165, w160) -> (resulting string=w168:string, error out=w167:errorcluster)  [unwired: 1 in]
        n90 = call <vilib>:"Error Cluster From Error Code.vi"("show call chain? (False)"=TRUE, "error in (no error)"=w167, "error message (\"\")"=w168, "error code (0)"=w169) -> ("error out"=w166:errorcluster)  [unwired: 5 in]
      }
      frame "Initialize Core Data" {
        # "Do not delete, rename, or modify this frame.\n(this is used to determine panel behavior on exit)"
        # "originally closed?"
        # "exe?"
        # "If panel starts closed or is an EXE, then close it when we exit"
        n91 = call <vilib>:"Add State(s) to Queue__jki_lib_state_machine.vi"("State(s) in (\"\")"=w182) -> ("States Out"=w181:string)  [unwired: 14 in]
        n92 = property class="VI"() -> ("Front Panel.Open"=w178:bool)  [unwired: 2 in, 2 out]
        n93 = Not(x=w178) -> (.not. x?=w175:bool)
        n94 = property class="App"() -> ("App.Kind"=w177:T19)  [unwired: 2 in, 2 out]
        n95 = Equal?(x=w177, y=T19."Run Time System" ("Application:Kind")) -> (x = y?=w174:bool)
        n96 = control-ref of="Current VI Reference"() -> (w171:refnum<vi>)
        n97 = Or(x=w175, y=w174) -> (x .or. y?=w172:bool)
        n98 = Bundle By Name(cluster=w173, "Core.Current VI Reference"=w171, "Core.Close Panel on Exit?"=w172) -> (w180:T22)
      }
      frame "Error Handler" {
        # "Unhandled Error -- Display it"
        # "Handle any errors here.\nYou can also output any states to clean-up after errors occur"
        # "Clear error"
        n99 = call <vilib>:"General Error Handler.vi"("error in (no error)"=w184) -> ()  [unwired: 10 in, 5 out]
        n100 = call <vilib>:"Add State(s) to Queue__jki_lib_state_machine.vi"("State(s) in Front (\"\")"="/* Post Error States", "State(s) in (\"\")"=w188) -> ("States Out"=w187:string)  [unwired: 13 in]
      }
      frame "Exit" {
        # "Do not put any code in this frame.\n(No errors that occur here will be handled.)"
        n101 = call <vilib>:"Add State(s) to Queue__jki_lib_state_machine.vi"("State(s) in (\"\")"=w193) -> ("States Out"=w192:string)  [unwired: 14 in]
      }
      frame "---------- Data ----------" {
        # "Do not put any code in this frame.\n(It is a separator no-op. You can make a copy of this frame to create a new Data frame)"
        n102 = call <vilib>:"Add State(s) to Queue__jki_lib_state_machine.vi"("State(s) in (\"\")"=w197) -> ("States Out"=w196:string)  [unwired: 14 in]
      }
      frame "Data: Initialize" {
        w198 = T23 {"STOP queue"=refnum, "SuperGUI ref"=refnum}  # SuperGUI
        w199 = T24 {"Current VI Reference"=refnum, "Close Panel on Exit?"=FALSE}  # Core
        w201 = TRUE  # Your Boolean data
        # "Initialize the shift-register data, here.\n(data names are defined by what you wire into the bundle function)"
        n103 = call <vilib>:"Add State(s) to Queue__jki_lib_state_machine.vi"("State(s) in (\"\")"=w205) -> ("States Out"=w204:string)  [unwired: 14 in]
        n104 = Bundle("Core"=w199, "Your Boolean data"=w201, "active cams"="active cams", "SuperGUI"=w198) -> (w203:T22)  [unwired: 1 in]
      }
      frame "Data: Cleanup" {
        # "Cleanup any data and references, here.\n(this is called automatically, by the Macro: Exit)"
        n105 = Unbundle By Name(w206) -> ("Core.Current VI Reference"=w209:refnum<vi>)
        n106 = call <vilib>:"Add State(s) to Queue__jki_lib_state_machine.vi"("State(s) in (\"\")"=w211) -> ("States Out"=w210:string)  [unwired: 14 in]
        n107 = Close Reference(reference=w209, error in (no error)=w208) -> (error out=w207:errorcluster)
      }
      frame "---------- UI ----------" {
        # "Do not put any code in this frame.\n(It is a separator no-op. You can make a copy of this frame to create a new UI frame)"
        n108 = call <vilib>:"Add State(s) to Queue__jki_lib_state_machine.vi"("State(s) in (\"\")"=w215) -> ("States Out"=w214:string)  [unwired: 14 in]
      }
      frame "UI: Initialize" {
        # "Initialize the User Interface, here.\n(this is called automatically, by the Macro: Init)"
        n109 = call <vilib>:"Add State(s) to Queue__jki_lib_state_machine.vi"("State(s) in (\"\")"=w222) -> ("States Out"=w221:string)  [unwired: 14 in]
        n110 = call <userlib>:"Fit VI window to Largest Dec__ogtk.vi"("error in (no error)"=w219) -> ("error out"=w218:errorcluster)  [unwired: 5 in, 1 out]
        n111 = for {
          tunnel: string[] ["Point Grey Camera", "Manta Camera", "Photometrics Cam", "Basler Camera"] -> [w224] mode=indexing
          tunnel: [w223] -> w216 mode=concatenating
          n112 = call "getDevices.vi"("Device Class"=w224) -> ("All Devices"=w223:string[])
        }
        n113 = property on="Select device" class="CmbBox"("Strings[]"=w216) -> ()  [unwired: 2 in, 2 out]
      }
      frame "UI: Get Device Name" {
        # "Initialize the User Interface, here.\n(this is called automatically, by the Macro: Init)"
        n114 = call <vilib>:"Add State(s) to Queue__jki_lib_state_machine.vi"("State(s) in (\"\")"=w230) -> ("States Out"=w229:string)  [unwired: 14 in]
        n115 = First Call?() -> (First Call?: T/F=w227:bool)
        n116 = case shown="True" w227 {
          tunnel: w226 -> [w231 w233]
          tunnel: [w231 w232] -> w225
          frame False {
          }
          frame True {
            n117 = disable-structure "Get Device name from control for vi mode\nand command line arg for exe" shown="RUN_TIME_ENGINE==True" {
              disable-tunnel: w233 -> [w234 w236]
              disable-tunnel: [w234 w235] -> w232
              frame condition #0 (active) {
              }
              frame condition #1 {
                n118 = control-ref of="This Application"() -> (w244:refnum<vi>)
                n119 = property class="App"(reference=w244) -> ("App.Args"=w243:string[])  [unwired: 1 in, 2 out]
                n120 = Index Array(array=w243, index #1=1 ("index")) -> (element #1=w237:string)  [unwired: 2 in, 2 out]
                n121 = Empty String/Path?(string/path=w237) -> (empty?=w241:bool)
                n122 = Concatenate Strings(w237, "_GUI ") -> (w239:string)
                n123 = case shown="False" w241 {
                  tunnel: w237 -> [w245 _]
                  frame False {
                    n124 = local write "GUIdevice 1"(w245) -> ()
                  }
                  frame True {
                  }
                }
                n125 = control-ref of="This VI"() -> (w240:refnum<vi>)
                n126 = property class="VI"(reference=w240, error in=w236, "Front Panel.Title"=w239) -> (error out=w235:errorcluster)  [unwired: 1 out]
              }
            }
          }
        }
      }
      frame "UI: Start SuperGUI" {
        # "create stop queue for supergui and its clones"
        # "x100 abort will be dependent on caller VI\nx80 abort will be independent of caller vi, this will abort vi when labview is closed."
        # "Start SuperGUI asynchronous way"
        n127 = vi-ref "GUI_Master_subvi_reentrant_queues.vi"() -> (w248:refnum<vi>)
        n128 = property class="VI"(reference=w248) -> ("Path"=w247:path)  [unwired: 1 in, 2 out]
        n129 = control-ref of="This Application"() -> (w254:refnum<vi>)
        n130 = Open VI Reference(type specifier VI Refnum (for type only)=refnum<vi> refnum, vi path=w247, options=256) -> (vi reference=w263:refnum<vi>, error out=w262:errorcluster)  [unwired: 3 in]
        n131 = Create User Event(user event datatype=T20 {"EventEnum"=enum."new data", "Device name"="Device name"} ("New Event"), error in=w250) -> (user event=w251:refnum<user-event>, error out=w257:errorcluster)
        "tcp data event" <- w251
        n132 = control-ref of="This VI"() -> (w253:refnum<vi>)
        n133 = register-events(w251) -> ()  [unwired: 2 in, 2 out]
        n134 = call "supergui create stop queue.vi"() -> ("STOP Queue out"=w259:refnum<queue>)  [unwired: 11 in]
        n135 = Current VI's Menubar() -> (w252:refnum<k9>)
        n136 = call-by-ref "Start Asynchronous Call"(reference=w263, error in=w262, "STOP Queue in"=w259, "This Application"=w254, 8:"error in (no error)"=w257, "tcp data event"=w251, "Caller menu reference"=w252, "Caller VI ref"=w253) -> (reference out=w246:refnum<vi>, error out=w249:errorcluster)  [unwired: 5 in, 1 out]
        n137 = Bundle By Name(cluster=w256, "SuperGUI.SuperGUI ref"=w246, "SuperGUI.STOP queue"=w259) -> (w255:T22)
        n138 = call <vilib>:"Add State(s) to Queue__jki_lib_state_machine.vi"("State(s) in (\"\")"=w265) -> ("States Out"=w264:string)  [unwired: 14 in]
      }
      frame "UI: Stop SuperGUI" {
        # "Stop Supergui Clone and wait until it exit properly"
        n139 = call <vilib>:"Add State(s) to Queue__jki_lib_state_machine.vi"("State(s) in (\"\")"=w273) -> ("States Out"=w272:string)  [unwired: 14 in]
        n140 = Unbundle By Name(w268) -> ("SuperGUI.SuperGUI ref"=w270:refnum<vi>, "SuperGUI.STOP queue"=w269:refnum<queue>)
        n141 = Release Queue(queue=w269, error in (no error)=w267) -> (error out=w271:errorcluster)  [unwired: 1 in, 2 out]
        n142 = call-by-ref "Wait On Asynchronous Call"(reference=w270, error in=w271) -> ("error out"=w266:errorcluster)  [unwired: 11 in, 2 out]
      }
      frame "UI: Cursor Set" {
        # "Argument"
        # "Set and Unset Cursor Busy.\n(Usage: \"UI: Cursor Set >> Busy|Idle\")"
        n143 = call <vilib>:"Add State(s) to Queue__jki_lib_state_machine.vi"("State(s) in (\"\")"=w279) -> ("States Out"=w278:string)  [unwired: 14 in]
        n144 = case shown="\"Idle\", Default" w274 {
          tunnel: w276 -> [w281 w283]
          tunnel: [w280 w282] -> w275
          frame "Idle", Default {
            n145 = call <vilib>:"Unset Busy.vi"("error in (no error)"=w281) -> ("error out"=w280:errorcluster)  [unwired: 10 in]
          }
          frame "Busy" {
            n146 = call <vilib>:"Set Busy.vi"("error in (no error)"=w283) -> ("error out"=w282:errorcluster)  [unwired: 9 in, 1 out]
          }
        }
      }
      frame "UI: Front Panel State" {
        # "Argument"
        # "Set Front Panel Open or Closed\n(Usage: \"UI: Front Panel State >> Open|Close\")"
        n147 = call <vilib>:"Add State(s) to Queue__jki_lib_state_machine.vi"("State(s) in (\"\")"=w290) -> ("States Out"=w289:string)  [unwired: 14 in]
        n148 = Unbundle By Name(w286) -> ("Core.Current VI Reference"=w285:refnum<vi>)
        n149 = case shown="\"Open\", Default" w284 {
          tunnel: w288 -> [w294 w307]
          tunnel: [w296 w308] -> w287
          tunnel: w285 -> [w295 w305]
          frame "Open", Default {
            n150 = property class="VI"(reference=w295, error in=w294) -> (reference out=w292:refnum<vi>, error out=w293:errorcluster, "Front Panel.Open"=w291:bool)
            n151 = case shown="False" w291 {
              tunnel: [w299 w302] -> w296
              tunnel: w293 -> [w298 w302]
              tunnel: w292 -> [w297 _]
              frame False {
                n152 = invoke class="VI" method="FP.Open"(reference=w297, error in=w298, "Activate"=TRUE, "State"=T21."Standard") -> (error out=w299:errorcluster)  [unwired: 1 in, 4 out]
              }
              frame True {
              }
            }
          }
          frame "Close" {
            n153 = property class="VI"(reference=w305, error in=w307) -> (reference out=w304:refnum<vi>, error out=w306:errorcluster, "Front Panel.Open"=w303:bool)
            n154 = case shown="True" w303 {
              tunnel: [w309 w312] -> w308
              tunnel: w306 -> [w309 w311]
              tunnel: w304 -> [_ w310]
              frame False {
              }
              frame True {
                n155 = invoke class="VI" method="FP.Close"(reference=w310, error in=w311) -> (error out=w312:errorcluster)  [unwired: 1 in, 2 out]
              }
            }
          }
        }
      }
      frame "---------- Macro ----------" {
        # "Do not put any code in this frame.\n(It is a separator no-op. You can make a copy of this frame to create a new Macro frame)"
        n156 = call <vilib>:"Add State(s) to Queue__jki_lib_state_machine.vi"("State(s) in (\"\")"=w316) -> ("States Out"=w315:string)  [unwired: 14 in]
      }
      frame "Macro: Initialize" {
        # "Initialization Macro\n(This is called once, when the VI starts)"
        n157 = call <vilib>:"Add State(s) to Queue__jki_lib_state_machine.vi"("State(s) in Front (\"\")"="Data: Initialize\nInitialize Core Data\nUI: Initialize\nUI: Get Device Name\nUI: Start SuperGUI\nUI: Front Panel State >> Open", "State(s) in (\"\")"=w321) -> ("States Out"=w320:string)  [unwired: 13 in]
      }
      frame "Macro: Exit" {
        # "Exit Macro\n(This is called once, when the VI exits)"
        n158 = Unbundle By Name(w328) -> ("Core.Close Panel on Exit?"=w327:bool)
        n159 = Select(t="UI: Front Panel State >> Close", s=w327, f="") -> (s? t:f=w324:string)
        n160 = call <vilib>:"Add State(s) to Queue__jki_lib_state_machine.vi"("State(s) in (\"\")"=w324, "State(s) at Back (\"\")"="Data: Cleanup\nExit") -> ("States Out"=w322:string)  [unwired: 13 in]
        n161 = call <vilib>:"Add State(s) to Queue__jki_lib_state_machine.vi"("State(s) in Front (\"\")"=w322, "State(s) in (\"\")"=w331) -> ("States Out"=w330:string)  [unwired: 13 in]
      }
      frame "---------- New Category ----------" {
        # "Template Separator\n(You can make a copy of, or modify, this frame)"
        n162 = call <vilib>:"Add State(s) to Queue__jki_lib_state_machine.vi"("State(s) in (\"\")"=w335) -> ("States Out"=w334:string)  [unwired: 14 in]
      }
      frame "New Category: 1" {
        # "Your code here.\n(You can make a copy of, or modify, this frame)"
        n163 = call <vilib>:"Add State(s) to Queue__jki_lib_state_machine.vi"("State(s) in (\"\")"=w339) -> ("States Out"=w338:string)  [unwired: 14 in]
      }
      frame "New Category: 2" {
        # "Your code here.\n(You can make a copy of, or modify, this frame)"
        n164 = call <vilib>:"Add State(s) to Queue__jki_lib_state_machine.vi"("State(s) in (\"\")"=w343) -> ("States Out"=w342:string)  [unwired: 14 in]
      }
    }
  }
